vi "Write Configiration Data.vi"(8 "error in (no error)":errorcluster, 10 "Configuration Settings":T1={"Signal type"=enum."Sine Wave", "Amplitude"=1.0, "Offset"=0.0, "Amplitude 2"=1.0, "Frequency"=10.0} {"Frequency" format="%0.2p"; "Amplitude 2" format="%.2p"; "Offset" format="%0.2p"; "Amplitude" format="%0.2p"}, 11 "Path":path) -> (0 "error out":errorcluster)   [LabVIEW 2022 SP3]
uses:
  controls/Configuration Settings.ctl
  <vilib>/Utility/config.llb/Write Key (Double).vi
  <vilib>/Utility/config.llb/Write Key (U32).vi
  <vilib>/Utility/config.llb/NI_LVConfig.lvlib
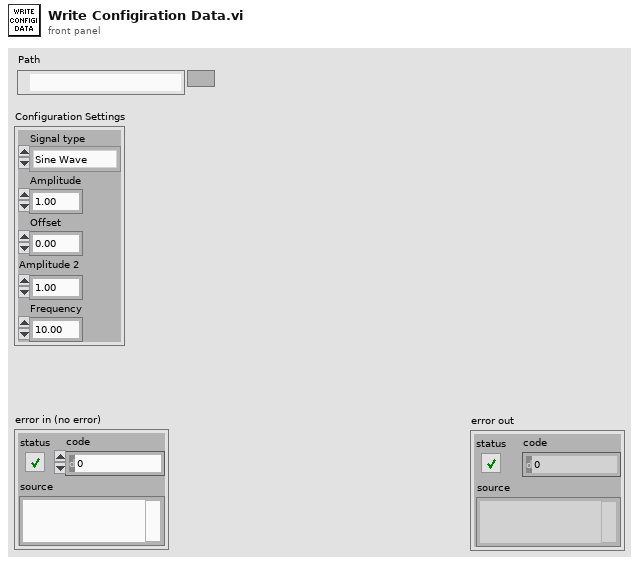
[diagram p1: front panel]
types:
  T1 = typedef "Configuration Settings.ctl" = cluster{"Signal type":enum16{"Sine Wave", "Triangle Wave", "Square Wave", "Sawtooth Wave"}, "Amplitude":dbl, "Offset":dbl, "Amplitude 2":dbl, "Frequency":dbl}
  T2 = enum16{"Sine Wave", "Triangle Wave", "Square Wave", "Sawtooth Wave"}
  T3 = typedef "NI_LVConfig.lvlib/Config Data RefNum.ctl" = refnum<k1>
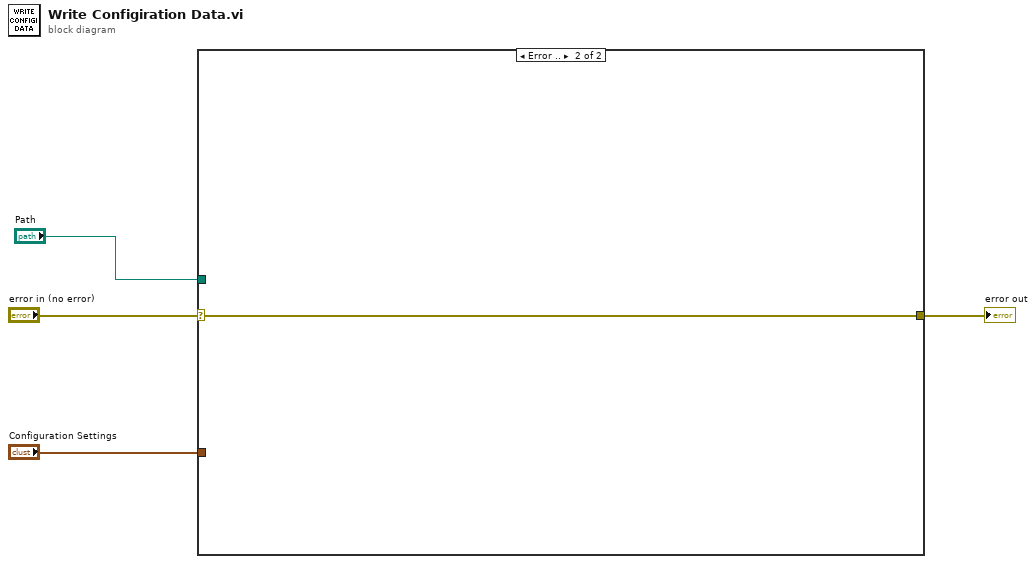
[diagram p0: block diagram]
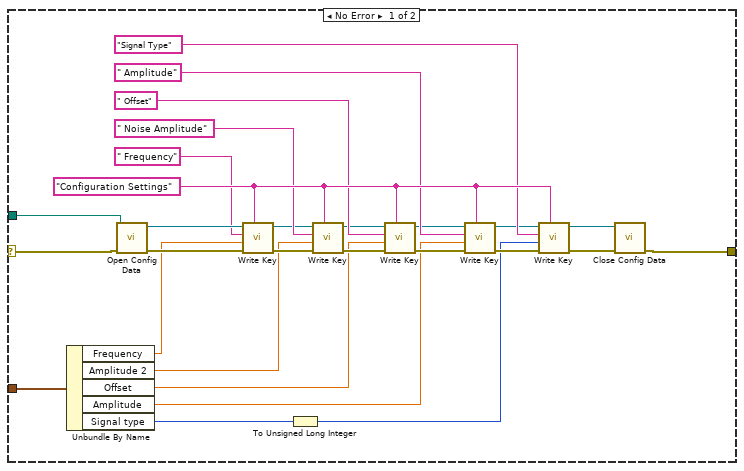
[diagram p2: hidden frame]
diagram:
  n1 = case shown="Error .." "error in (no error)" {
    selector: "error in (no error)" -> [w18 w33]
    tunnel: [w11 w33] -> w3
    tunnel: "Path" -> [w31 _]
    tunnel: "Configuration Settings" -> [w32 _]
    frame No Error {
      w29 = "Configuration Settings" ("section")
      n2 = Unbundle By Name(w32) -> ("Frequency"=w10:dbl, "Amplitude 2"=w9:dbl, "Offset"=w8:dbl, "Amplitude"=w7:dbl, "Signal type"=w5:T2)
      n3 = call <vilib>:"Open Config Data.vi"("error in (no error)"=w18, "configuration file path"=w31) -> ("error out"=w17:errorcluster, "refnum"=w30:T3)  [unwired: 7 in, 1 out]
      n4 = call-poly <vilib>:"Write Key.vi"("section"=w29, "error in (no error)"=w17, "value"=w10, "key"=" Frequency", "refnum"=w30) -> ("error out"=w16:errorcluster, "refnum out"=w23:T3)  [unwired: 4 in, 1 out]
      n5 = To Unsigned Long Integer(number=w5) -> (unsigned 32bit integer=w6:u32)
      n6 = call-poly <vilib>:"Write Key.vi"("section"=w29, "error in (no error)"=w16, "value"=w9, "key"=" Noise Amplitude", "refnum"=w23) -> ("error out"=w15:errorcluster, "refnum out"=w22:T3)  [unwired: 4 in, 1 out]
      n7 = call-poly <vilib>:"Write Key.vi"("section"=w29, "error in (no error)"=w15, "value"=w8, "key"=" Offset", "refnum"=w22) -> ("error out"=w14:errorcluster, "refnum out"=w21:T3)  [unwired: 4 in, 1 out]
      n8 = call-poly <vilib>:"Write Key.vi"("section"=w29, "error in (no error)"=w14, "value"=w7, "key"=" Amplitude", "refnum"=w21) -> ("error out"=w13:errorcluster, "refnum out"=w20:T3)  [unwired: 4 in, 1 out]
      n9 = call-poly <vilib>:"Write Key.vi"("section"=w29, "error in (no error)"=w13, "value"=w6, "key"="Signal Type", "refnum"=w20) -> ("error out"=w12:errorcluster, "refnum out"=w19:T3)  [unwired: 4 in, 1 out]
      n10 = call <vilib>:"Close Config Data.vi"("error in (no error)"=w12, "refnum"=w19) -> ("error out"=w11:errorcluster)  [unwired: 8 in, 1 out]
    }
    frame Error {
    }
  }
  "error out" <- w3
